vi "AFT Set Coefficients.vi"   [LabVIEW 2017, in "NI_AdaptiveFilter.lvlib"]
doc: "Sets the coefficients of an adaptive filter that you create with the least mean squares (LMS) or recursive least squares (RLS) algorithms. You must manually select the polymorphic instance you want to use."
uses:
  <vilib>/addons/Adaptive Filters/NI_AdaptiveFilter.lvlib
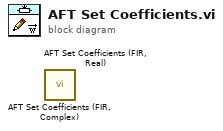
[diagram p0: block diagram]
diagram:
  n1 = call <vilib>:"AFT Set Coefficients (FIR, Complex).vi"() -> ()  [unwired: 10 in, 2 out]
  n2 = call <vilib>:"AFT Set Coefficients (FIR, Real).vi"() -> ()  [unwired: 10 in, 2 out]
